vi "DataLog_CleanString.vi"(11 "Notes in":string) -> (3 "Notes out":string)   [LabVIEW 2014, in "ShhgDataLogging.lvlib"]
uses:
  ShhgDataLogging.lvlib
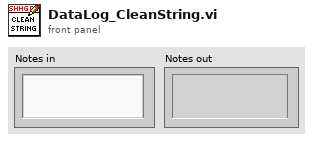
[diagram p1: front panel]
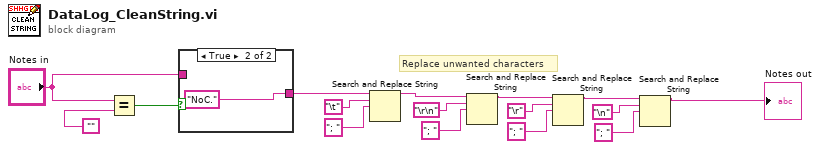
[diagram p0: block diagram]
diagram:
  # "Replace unwanted characters"
  n1 = Equal?(x="Notes in", y="") -> (x = y?=w16:bool)
  n2 = case shown="True" w16 {
    tunnel: [w17 "NoC."] -> w11
    tunnel: "Notes in" -> [w17 _]
    frame False {
    }
    frame True {
    }
  }
  n3 = Search and Replace String(input string=w11, search string="\t", replace string="; " ("replace string (\"\")")) -> (result string=w4:string)  [unwired: 5 in, 3 out]
  n4 = Search and Replace String(input string=w4, search string="\r\n", replace string="; " ("replace string (\"\")")) -> (result string=w3:string)  [unwired: 5 in, 3 out]
  n5 = Search and Replace String(input string=w3, search string="\r", replace string="; " ("replace string (\"\")")) -> (result string=w2:string)  [unwired: 5 in, 3 out]
  n6 = Search and Replace String(input string=w2, search string="\n", replace string="; " ("replace string (\"\")")) -> (result string=→"Notes out":string)  [unwired: 5 in, 3 out]
